vi "DSF.Engine.Pointer.DBL.New.vi"(8 "error in (no error)":errorcluster, 11 "channel count":u64) -> (0 "error out":errorcluster, 3 "DBL Pointer out":refnum<class "DSF.Engine.Pointer.DBL.lvclass">)   [LabVIEW 2017, in "DSF.Engine.lvlib" / "DSF.Engine.Pointer.DBL.lvclass"]
uses:
  DSF.Engine.Pointer.DBL.lvclass
  C:/github/data-sharing-framework/dsf core/Built/Memory/Memory Manager.lvlibp/1abvi3w/vi.lib/National Instruments/Memory Manager/Classes/Pointer/Memory.Pointer.lvclass
  DSF.Engine.Pointer.DBL.lvclass/DSF.Engine.Pointer.DBL.ctl
  Built/Memory/Memory Manager.lvlibp/1abvi3w/vi.lib/National Instruments/Memory Manager/Classes/Pointer/Memory.Pointer.New.8B.vi
  Built/Memory/Memory Manager.lvlibp/1abvi3w/vi.lib/National Instruments/Memory Manager/Classes/Pointer/Memory.Pointer.lvclass
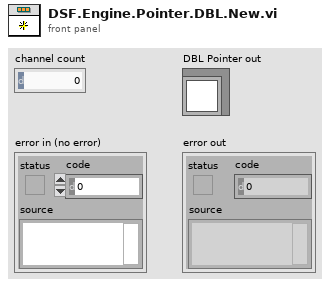
[diagram p1: front panel]
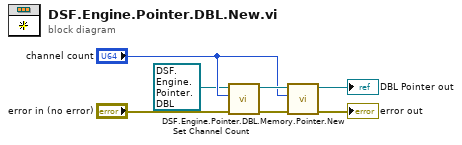
[diagram p0: block diagram]
diagram:
  n1 = call "DSF.Engine.Pointer.DBL.Set Channel Count.vi"("channel count"="channel count", "DBL Buffer in"=refnum<class "DSF.Engine.Pointer.DBL.lvclass"> refnum) -> ("DBL Buffer out"=w6:refnum<class "DSF.Engine.Pointer.DBL.lvclass">)  [unwired: 9 in]
  n2 = call-poly "Memory.Pointer.New.vi"("error in (no error)"="error in (no error)", "count (1)"="channel count", "Pointer type"=w6) -> ("error out"=→"error out":errorcluster, "Pointer"=→"DBL Pointer out":refnum<class "DSF.Engine.Pointer.DBL.lvclass">)  [unwired: 7 in]
